vi "Add SRs.vi"(8 "error in":errorcluster, 9 "entered SRs in":i32[](array[numeric]), 11 "Data Loop Data in":T1) -> (0 "error out":errorcluster, 3 "Data Loop Data out":T1)   [LabVIEW 2018]
uses:
  Type Defs/Screenpop Loop Data.ctl
  Support/Message Queue/Message Cluster.ctl
  Support/Message Queue/Message Queue.lvlib
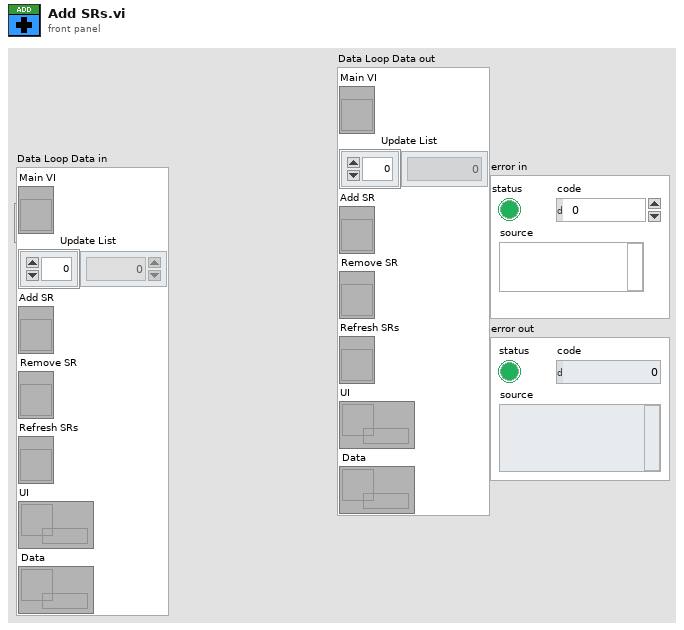
[diagram p1: front panel]
types:
  T1 = typedef "Screenpop Loop Data.ctl" = cluster{"Main VI":refnum<vi>, "Update List":i32[], "Add SR":refnum<vi>, "Remove SR":refnum<vi>, "Refresh SRs":refnum<vi>, "UI":refnum<queue>, "Data":refnum<queue>}
  T2 = typedef "SR Cluster.ctl" = cluster{"Color":u32, "SR Number":i32, "SR Status":T3, "Name":string, "Summary":string, "Last Updated":timestamp, "SR Type":string, "Service Level":string, "Days Open":dbl, "Creation Date":timestamp, "Owner":string}
  T3 = typedef "SR Status.ctl" = enum16{"Caller Abandoned", "Created in Error", "Expired", "Forum Resolved AE", "Forum Resolved Customer", "IN WORK", "IN WORK Collab with AES", "IN WORK Collab with PSE", "IN WORK Collab with SE", "IN WORK Customer Added Note", "IN WORK Escalation", "IN WORK Wait on Customer", "Open", "Potentially Resolved", "Presumed Resolved", "RMA Approved for Return", "RMA Closed", "RMA Closed - DOA", "RMA In Progress", "RMA Open", "RMA Waiting on Customer", "Resolved", "Passed Off"}
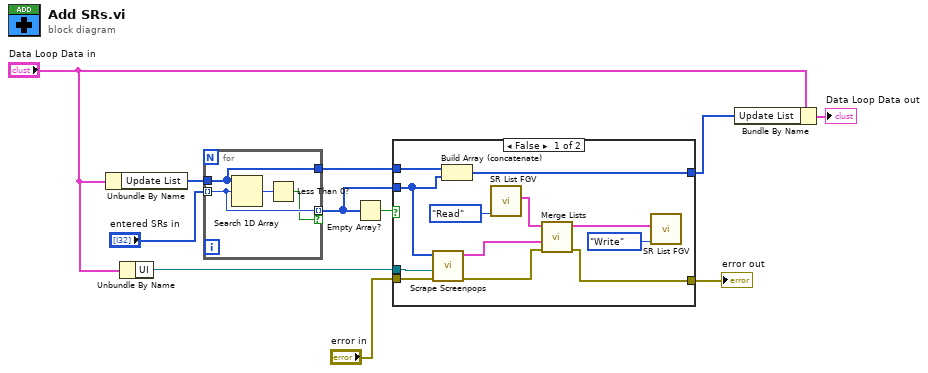
[diagram p0: block diagram]
diagram:
  n1 = Unbundle By Name("Data Loop Data in") -> ("Update List"=w11:i32[])
  n2 = Unbundle By Name("Data Loop Data in") -> ("UI"=w1:refnum<queue>)
  n3 = for {
    tunnel: "entered SRs in" -> [w14] mode=indexing
    tunnel: w11 -> [w12]
    tunnel: [w14] -> w7 mode=indexing if=w13
    tunnel: [w12] -> w6
    n4 = Search 1D Array(1D array=w12, element=w14) -> (index of element=w15:i32)  [unwired: 1 in]
    n5 = Less Than 0?(x=w15) -> (x < 0?=w13:bool)
  }
  n6 = Empty Array?(array=w7) -> (empty?=w8:bool)
  n7 = case shown="False" w8 {
    tunnel: w7 -> [w23 _]
    tunnel: [w24 w29] -> w5
    tunnel: w6 -> [w27 w29]
    tunnel: "error in" -> [w22 w28]
    tunnel: [w20 w28] -> w3
    tunnel: w1 -> [w16 _]
    frame False {
      n8 = call "Scrape Screenpops.vi"("error in"=w22, "UI"=w16, "SR number list in"=w23) -> ("error out"=w21:errorcluster, "sr clusters out"=w19:T2[])  [unwired: 7 in]
      n9 = Build Array (concatenate)(w27, w23) -> (w24:i32[])
      n10 = call "SR List FGV.vi"("Operation"=enum16{"Initialize", "Write", "Read", "Clear"}."Read") -> ("list out"=w26:T2[])  [unwired: 9 in, 1 out]
      n11 = call "Merge Lists.vi"("error in"=w21, "new list in"=w19, "list in"=w26) -> ("error out"=w20:errorcluster, "list out"=w17:T2[])  [unwired: 7 in]
      n12 = call "SR List FGV.vi"("Operation"=enum16{"Initialize", "Write", "Read", "Clear"}."Write", "list in"=w17) -> ()  [unwired: 8 in, 2 out]
    }
    frame True {
    }
  }
  "error out" <- w3
  n13 = Bundle By Name(cluster="Data Loop Data in", "Update List"=w5) -> (→"Data Loop Data out":T1)
